vi "Calibrate Adc Table Data Query.vi"(8 "error in":errorcluster, 9 "Table Index":i32 format="%.0g", 10 "Input Channel":i32(ring) items=["Input Channel 1", "Input Channel 2", "Input Channel 3", "Input Channel 4"], 11 "Instrument Handle In":i32) -> (0 "error out":errorcluster, 1 "ADC Code":u16, 2 "Scale Factor":u16, 3 "Instrument Handle Out":i32)   [LabVIEW 8.6, in "ZTScopeM.lvlib"]
doc: "Query the instrument's ADC calibration codes. See the instrument calibration manual for more information."
uses:
  ZTScopeM.lvlib
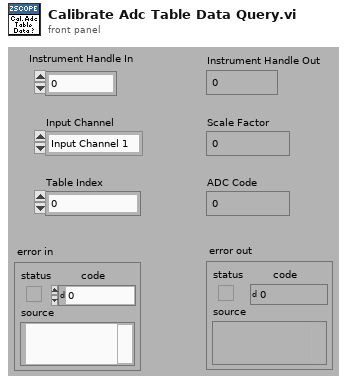
[diagram p1: front panel]
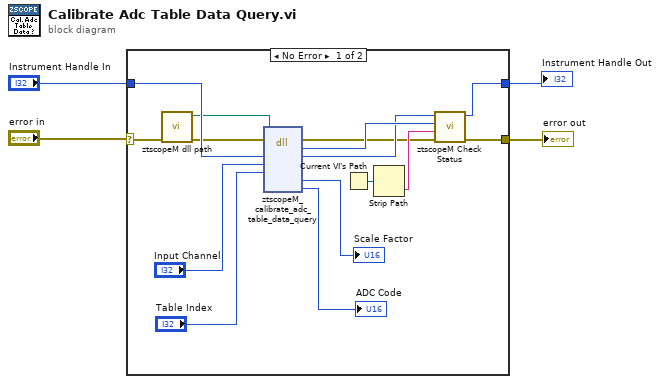
[diagram p0: block diagram]
diagram:
  n1 = case shown="No Error" "error in" {
    selector: "error in" -> [w8 w21]
    tunnel: [w14 w21] -> w1
    tunnel: "Instrument Handle In" -> [w19 w20]
    tunnel: [w13 w20] -> w3
    frame #0 {
      n2 = call "ztscopeM dll path.vi"("error in (no error)"=w8) -> ("error out"=w6:errorcluster, "<instrument>.dll path"=w7:path)  [unwired: 9 in]
      n3 = dll-call lib="C:/Program Files (x86)/National Instruments/LabVIEW 2013/instr.lib/ztscopem/ztscopeM.dll" fn="ztscopeM_calibrate_adc_table_data_query"(path in=w7, error in=w6, "instrumentHandle"=w19, "channel"="Input Channel", "tableIndex"="Table Index") -> (error out=w5:errorcluster, w16:i32, "instrumentHandle"=w15:i32, "scaleFactor"=→"Scale Factor":u16, "adcCode"=→"ADC Code":u16)  [unwired: 5 in, 1 out]
      n4 = Current VI's Path() -> (path=w18:path)
      n5 = Strip Path(path=w18) -> (name=w17:string)  [unwired: 1 out]
      n6 = call "ztscopeM Check Status.vi"("error in"=w5, "name of VI"=w17, "status (return code)"=w16, "instrument handle in"=w15) -> ("error out"=w14:errorcluster, "instrument handle out"=w13:i32)  [unwired: 2 in]
    }
    frame #1 {
    }
  }
  "Instrument Handle Out" <- w3
  "error out" <- w1
